vi "TSM Relay Pins to Sessions.vi"(0 "TSM context":T2, 5 "Relay Pins":string[](array[string]), 9 "Site Numbers":i32[](array[numeric]), 11 "error in":errorcluster) -> (4 "TSM Relay":T1={"TSM context"=refnum, "Pin Query Context"=refnum, "TSM Site Numbers"=[], "SSC Relay"=[], "Unfiltered Pins"=[], "Filtered Pins"=[], "Filtered Pins Info"={"Unfiltered Pins Count"=3, "Locations"=[], "Lengths"=[]}}, 15 "error out":errorcluster)   [LabVIEW 2019]
doc: "Populates the TSM Relay cluster for the specified pin(s) and pin group(s). \n\nUse this VI in place of TSM Relay Pins to Sessions VI when optimizing for test time - this allows users to call Get Site Numbers only once in their code module and reduce the number of TSM context calls."
uses:
  <vilib>/NI_TestStand_SemiconductorModule/NI_TestStand_Semiconductor_Module.lvlibp/PinMap/General/SemiconductorModuleContext.ctl
  SubVIs/TSM SSC Relay.ctl
  <vilib>/NI_TestStand_SemiconductorModule/NI_TestStand_Semiconductor_Module.lvlibp/PinMap/PinQueryContext/MultiplePinMultipleSessionQueryContext/MultiplePinMultipleSessionQueryContext.lvclass
  SSC/SSC Relay.ctl
  SubVIs/TSM Filtered Pins Info.ctl
  Pin Map/TSM Relay Instrument Type ID.vi
  Pin Map/TSM Relay PinTypeInfo.vi
  <vilib>/NI_TestStand_SemiconductorModule/NI_TestStand_Semiconductor_Module.lvlibp/PinMap/Advanced/GetRelaysInRelayGroup(s).vi
  <vilib>/NI_TestStand_SemiconductorModule/NI_TestStand_Semiconductor_Module.lvlibp/PinMap/Advanced/GetRelaysInRelayGroups.vi
  <vilib>/NI_TestStand_SemiconductorModule/NI_TestStand_Semiconductor_Module.lvlibp/PinMap/Advanced/Custom Instruments/GetSessionDataPolymorphic.vi
  <vilib>/NI_TestStand_SemiconductorModule/NI_TestStand_Semiconductor_Module.lvlibp/PinMap/Advanced/Custom Instruments/GetSessionData.vi
  <vilib>/NI_TestStand_SemiconductorModule/NI_TestStand_Semiconductor_Module.lvlibp
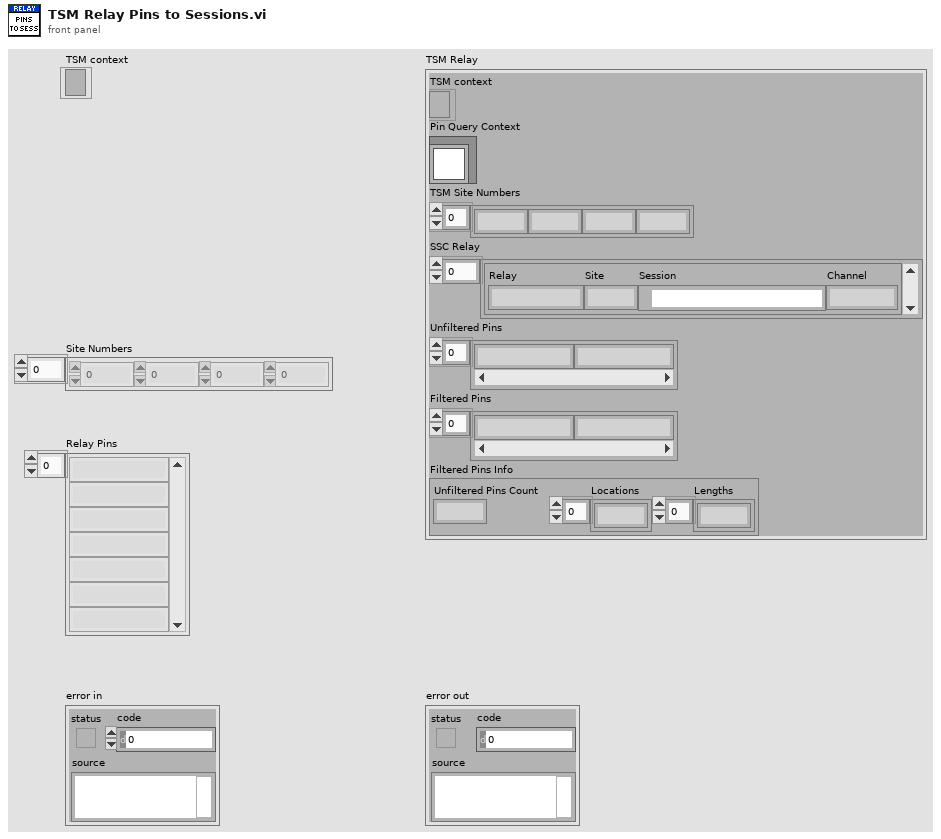
[diagram p1: front panel]
types:
  T1 = typedef "TSM SSC Relay.ctl" = cluster{"TSM context":T2, "Pin Query Context":refnum<class "MultiplePinMultipleSessionQueryContext.lvclass">, "TSM Site Numbers":i32[], "SSC Relay":T3[], "Unfiltered Pins":string[], "Filtered Pins":string[], "Filtered Pins Info":T4}
  T2 = typedef "NI_TestStand_Semiconductor_Module.lvlibp/SemiconductorModuleContext.ctl" = refnum<k7>
  T3 = typedef "SSC Relay.ctl" = cluster{"Relay":string, "Site":i32, "Session":refnum<k15>, "Channel":string}
  T4 = typedef "TSM Filtered Pins Info.ctl" = cluster{"Unfiltered Pins Count":i32, "Locations":i32[], "Lengths":i32[]}
  T5 = cluster{"Pin":string, "Number Of Sites":i32, "instrument handle out":refnum<k15>, "Channel List":string}[]
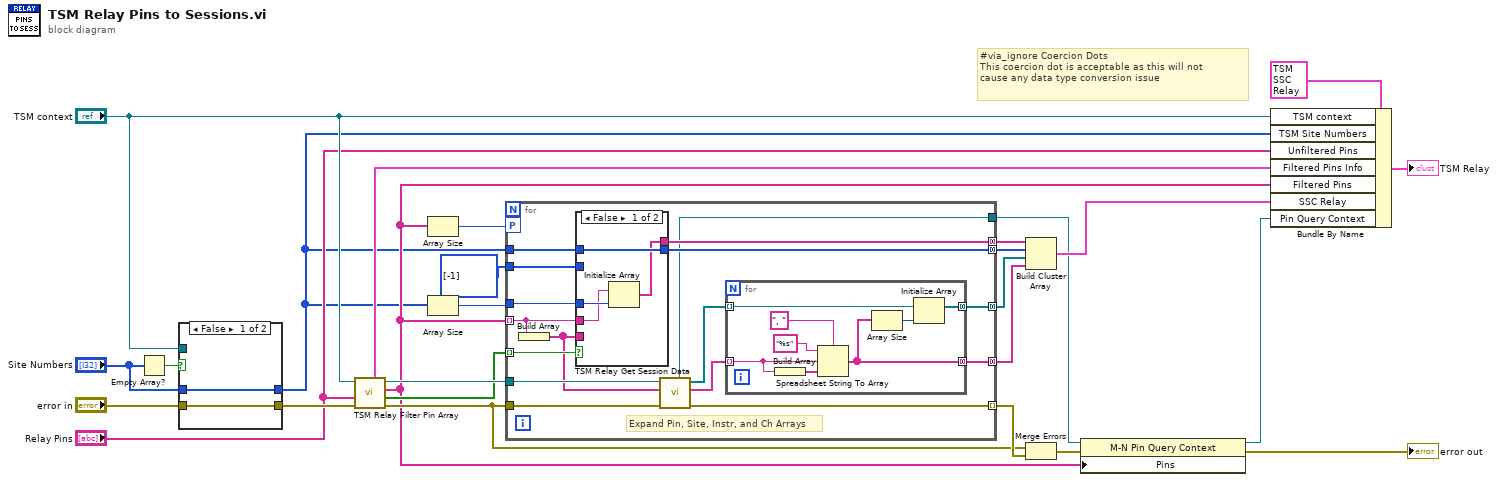
[diagram p0: block diagram]
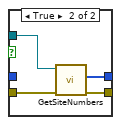
[diagram p3: hidden frame]
diagram:
  # "#via_ignore Coercion Dots\nThis coercion dot is acceptable as this will not\ncause any data type conversion issue"
  n1 = Empty Array?(array="Site Numbers") -> (empty?=w3:bool)
  n2 = case shown="False" w3 {
    tunnel: "Site Numbers" -> [w29 _]
    tunnel: [w29 w32] -> w4
    tunnel: "TSM context" -> [_ w33]
    tunnel: "error in" -> [w28 w31]
    tunnel: [w28 w30] -> w27
    frame False {
    }
    frame True {
      n3 = call <vilib>:"GetSiteNumbers.vi"("error in (no error)"=w31, "Semiconductor Module Context"=w33) -> ("error out"=w30:errorcluster, "Site Numbers"=w32:i32[])  [unwired: 6 in, 2 out]
    }
  }
  n4 = call "TSM Relay Filter Pin Array.vi"("error in"=w27, "Pins"="Relay Pins", "TSM context in"="TSM context") -> ("error out"=w9:errorcluster, "Is System Pin"=w21:bool[], "Filtered Pins Array"=w7:string[], "TSM context out"=w23:T2, "Filtered Pins Info"=w11:T4)  [unwired: 4 in]
  n5 = Array Size(array=w7) -> (size(s)=w6:i32)
  n6 = Array Size(array=w4) -> (size(s)=w5:i32)
  n7 = for {
    tunnel: w23 -> [w47]
    tunnel: w7 -> [w35] mode=indexing
    tunnel: [w44] -> w17 mode=concatenating
    tunnel: [w43] -> w16 mode=concatenating
    tunnel: w21 -> [w42] mode=indexing
    tunnel: w5 -> [w38]
    tunnel: w4 -> [w40]
    tunnel: [w41] -> w20 mode=concatenating
    tunnel: [w39] -> w19 mode=concatenating
    tunnel: [w37] -> w13
    workers-P: w6 -> [_]
    tunnel: w9 -> [w49]
    tunnel: [w48] -> w18 mode=indexing
    tunnel: i32[] [-1] ("Number Of Sites") -> [w36]
    # "Expand Pin, Site, Instr, and Ch Arrays"
    n8 = Build Array(w35) -> (w34:string[])
    n9 = case shown="False" w42 {
      tunnel: w35 -> [w50 _]
      tunnel: [w52 w54] -> w41
      tunnel: w40 -> [w53 _]
      tunnel: [w53 w55] -> w39
      tunnel: w38 -> [w51 _]
      tunnel: w36 -> [_ w55]
      tunnel: w34 -> [_ w54]
      frame False {
        n10 = Initialize Array(w50, w51) -> (w52:string[])
      }
      frame True {
      }
    }
    n11 = call "TSM Relay Get Session Data.vi"("error in"=w49, "Pins"=w34, "TSM context"=w47) -> ("error out"=w48:errorcluster, "Channel Lists"=w46:string[], "Instrument Sessions"=w45:refnum<k15>[], "Pin Query Context"=w37:refnum<class "MultiplePinMultipleSessionQueryContext.lvclass">)  [unwired: 4 in, 1 out]
    n12 = for {
      tunnel: w46 -> [w61] mode=indexing
      tunnel: [w57] -> w44 mode=concatenating
      tunnel: w45 -> [w59] mode=indexing
      tunnel: [w58] -> w43 mode=concatenating
      n13 = Build Array(w61) -> (w60:string[])
      n14 = Spreadsheet String To Array(delimiter (Tab)=", ", format string="%s", spreadsheet string=w61, array type (2D Dbl)=w60) -> (array=w57:string[])
      n15 = Array Size(array=w57) -> (size(s)=w56:i32)
      n16 = Initialize Array(w59, w56) -> (w58:refnum<k15>[])
    }
  }
  n17 = Build Cluster Array(w20, w19, w16, w17) -> (w15:T5)
  n18 = Merge Errors(w9, w18) -> (w10:errorcluster)
  n19 = property class="M-N Pin Query Context"(reference=w13, error in=w10, "Pins"=w7) -> (reference out=w12:refnum<class "MultiplePinMultipleSessionQueryContext.lvclass">, error out=→"error out":errorcluster)
  n20 = Bundle By Name(cluster=T1 {"TSM context"=refnum, "Pin Query Context"=refnum, "TSM Site Numbers"=[], "SSC Relay"=[], "Unfiltered Pins"=[], "Filtered Pins"=[], "Filtered Pins Info"={"Unfiltered Pins Count"=3, "Locations"=[], "Lengths"=[]}} ("Relay - Sessions Info"), "TSM context"="TSM context", "TSM Site Numbers"=w4, "Unfiltered Pins"="Relay Pins", "Filtered Pins Info"=w11, "Filtered Pins"=w7, "SSC Relay"=w15, "Pin Query Context"=w12) -> (→"TSM Relay":T1)
